vi "CRIOhack.vi"() -> ()   [LabVIEW 2010]
panel:
  out "data":waveform(dbl)[](array[waveform])
  out "channel name(s) out":string[](array[string])
  out "error out":errorcluster
  in  "file path":path
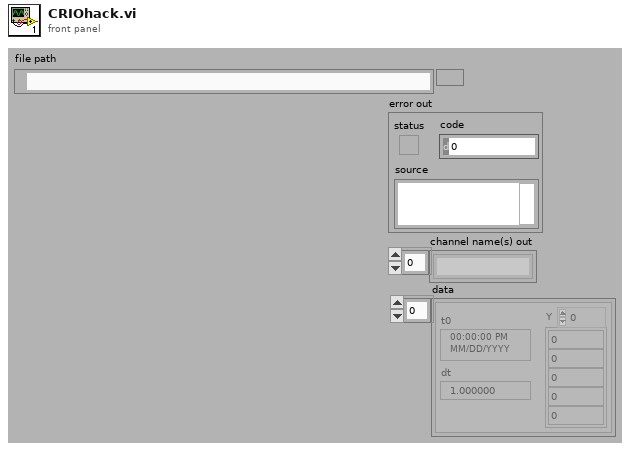
[diagram p1: front panel]
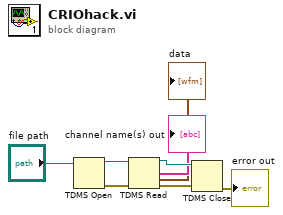
[diagram p0: block diagram]
diagram:
  n1 = TDMS Open(11:"file path") -> (0:w6:errorcluster, 3:w7:refnum<k34>)  [unwired: 5 in]
  n2 = TDMS Read(0:w7, 11:w6) -> (4:w4:refnum<k34>, 8:→"channel name(s) out":string[], 10:→"data":waveform(dbl)[], 15:w5:errorcluster)  [unwired: 5 in, 2 out]
  n3 = TDMS Close(8:w5, 11:w4) -> (0:→"error out":errorcluster)  [unwired: 1 out]
